vi "Open_Instr.vi"(8 "error in (no error)":errorcluster caption="entrée d'erreur (pas d'erreur)", 11 "Class Relay_Board en entrée":refnum<class "Class Instrument Relay_Board.lvclass">) -> (0 "error out":errorcluster caption="sortie d'erreur", 3 "Class Relay_Board en Sortie":refnum<class "Class Instrument Relay_Board.lvclass">)   [LabVIEW 2020, in "Library Instrument & Equipement.lvlib" / "Library Instruments.lvlib" / "Class Instrument Relay_Board.lvclass"]
uses:
  Class Instrument Relay_Board.lvclass
  Class Instrument Relay_Board.lvclass/Class Instrument Relay_Board.ctl
  Instrument (Default)/Class Instrument (Default).lvclass
  Relay_Board/Relay_Board (Default)/Class Relay_Board (Default).lvclass
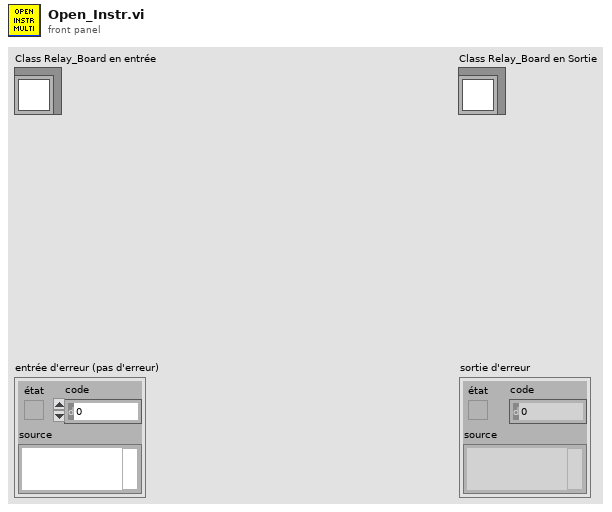
[diagram p1: front panel]
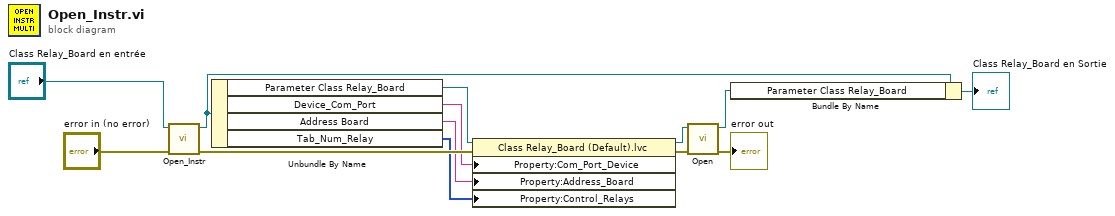
[diagram p0: block diagram]
diagram:
  n1 = call-parent "Open_Instr.vi"("error in (no error)"="error in (no error)", "Class Multimeter (Default) en entrée"="Class Relay_Board en entrée") -> ("error out"=w10:errorcluster, "Class Multimeter (Default) en sortie"=w5:refnum<class "Class Instrument Relay_Board.lvclass">)  [unwired: 8 in]
  n2 = Unbundle By Name(w5) -> ("Parameter Class Relay_Board"=w8:refnum<class "Class Relay_Board (Default).lvclass">, "Device_Com_Port"=w7:string, "Address Board"=w6:string, "Tab_Num_Relay"=w2:u8[])
  n3 = property class="Class Relay_Board (Default).lvc"(reference=w8, error in=w10, "Property:Com_Port_Device"=w7, "Property:Address_Board"=w6, "Property:Control_Relays"=w2) -> (reference out=w3:refnum<class "Class Relay_Board (Default).lvclass">, error out=w9:errorcluster)
  n4 = call-dynamic "Open.vi"("error in (no error)"=w9, "Class Relay_Board (Default) en entrée"=w3) -> ("error out"=→"error out":errorcluster, "Class Relay_Board (Default) en sortie"=w1:refnum<class "Class Relay_Board (Default).lvclass">)  [unwired: 8 in]
  n5 = Bundle By Name(cluster=w5, "Parameter Class Relay_Board"=w1) -> (→"Class Relay_Board en Sortie":refnum<class "Class Instrument Relay_Board.lvclass">)
